vi "FTW-Tag-Get.vi"(0 "FTW Actor Connector In":refnum<class "FTW-ActorConnector.lvclass">, 5 "Tag Object":string, 11 "error in (no error)":errorcluster) -> (4 "FTW Actor Connector":refnum<class "FTW-ActorConnector.lvclass">, 6 "Response":string, 14 "Roundtrip Time":dbl format="%.6f sec", 15 "error out":errorcluster)   [LabVIEW 2015]
uses:
  Connector/FTW-ActorConnector.lvclass
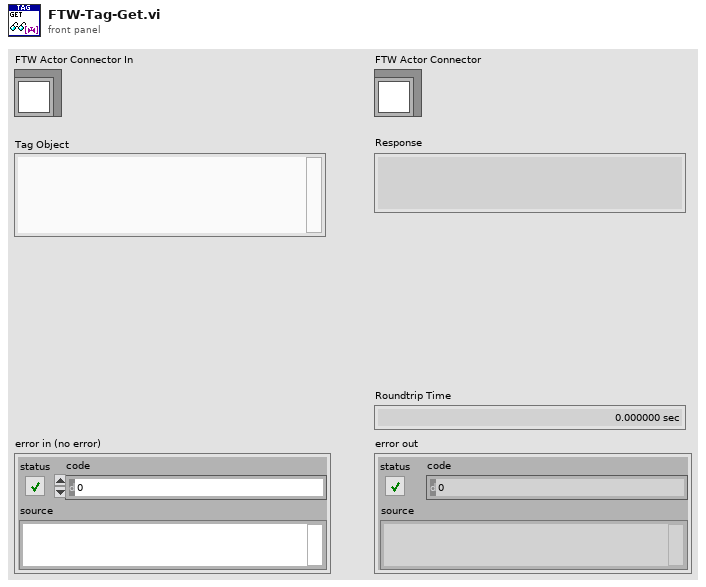
[diagram p1: front panel]
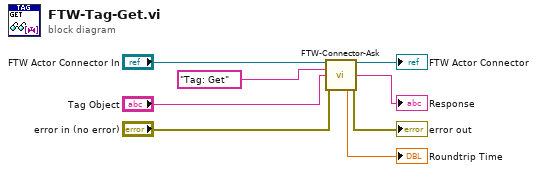
[diagram p0: block diagram]
diagram:
  n1 = call "FTW-Connector-Ask.vi"("FTW Actor Connector"="FTW Actor Connector In", "Request Header"="Tag: Get", "Request Body"="Tag Object", "error in"="error in (no error)") -> ("FTW Actor Connector out"=→"FTW Actor Connector":refnum<class "FTW-ActorConnector.lvclass">, "Response Body"=→"Response":string, "Roundtrip Time"=→"Roundtrip Time":dbl, "error out"=→"error out":errorcluster)  [unwired: 6 in, 2 out]
